vi "大富翁.vi"() -> ()   [LabVIEW 2014] (continued)
                  }
                  frame 2 {
                    n3261 = local read "玩家二財產"() -> (w2676:dbl)
                  }
                  frame 3 {
                    n3262 = local read "玩家三財產"() -> (w2677:dbl)
                  }
                  frame 4 {
                    n3263 = local read "玩家四財產"() -> (w2678:dbl)
                  }
                }
                n3264 = Equal?(x=w2622, y=w2646) -> (x = y?=w2645:bool)
                n3265 = local read "嘉義縣所有"() -> (w2623:u32)
                n3266 = local read "23旅4"() -> (w2624:bool)
                n3267 = local read "23旅3"() -> (w2625:bool)
                n3268 = local read "23旅2"() -> (w2626:bool)
                n3269 = local read "23旅1"() -> (w2627:bool)
                n3270 = local read "23房4"() -> (w2628:bool)
                n3271 = local read "23房3"() -> (w2629:bool)
                n3272 = local read "23房2"() -> (w2630:bool)
                n3273 = local read "23房1"() -> (w2631:bool)
                n3274 = call "房子數量.vi"("房子 1"=w2631, "房子 2"=w2630, "房子 3"=w2629, "房子 4"=w2628, "旅館 1"=w2627, "旅館 2"=w2626, "旅館 3"=w2625, "旅館 4"=w2624) -> ("房子數"=w2644:dbl, "旅館數"=w2643:dbl)  [unwired: 18 in]
                n3275 = call "顏色轉數字.vi"("顏色數字"=w2623) -> ("數字"=w2633:dbl)  [unwired: 2 in]
                n3276 = case shown="1, Default" w2633 {
                  tunnel: [w2651 w2652 w2653 w2654] -> w2637
                  frame 1, Default {
                    n3277 = local read "玩家一財產"() -> (w2651:dbl)
                  }
                  frame 2 {
                    n3278 = local read "玩家二財產"() -> (w2652:dbl)
                  }
                  frame 3 {
                    n3279 = local read "玩家三財產"() -> (w2653:dbl)
                  }
                  frame 4 {
                    n3280 = local read "玩家四財產"() -> (w2654:dbl)
                  }
                }
                n3281 = call "走到地.vi"("房子數量"=w2644, "自己的地?"=w2645, "旅館數量"=w2643, "編號"=w2642, "走到人財產"=w2641) -> ("走到人-?"=w2640:dbl, "蓋第幾棟"=w2638:dbl, "地主+?"=w2636:dbl, "破產?"=w2632:bool)
                n3282 = Subtract(x=w2641, y=w2640) -> (x-y=w2639:dbl)
                n3283 = Add(x=w2636, y=w2637) -> (x+y=w2634:dbl)
                n3284 = case shown="1, Default" w2633 {
                  tunnel: w2634 -> [w2647 w2648 w2649 w2650]
                  frame 1, Default {
                    n3285 = local write "玩家一財產"(w2647) -> ()
                  }
                  frame 2 {
                    n3286 = local write "玩家二財產"(w2648) -> ()
                  }
                  frame 3 {
                    n3287 = local write "玩家三財產"(w2649) -> ()
                  }
                  frame 4 {
                    n3288 = local write "玩家四財產"(w2650) -> ()
                  }
                }
                n3289 = case shown="7" w2638 {
                  frame 0, Default {
                  }
                  frame 1 {
                    n3290 = flat-sequence {
                      frame #0 {
                        n3291 = local write "23房1"(TRUE ("1房1")) -> ()
                      }
                      frame #1 {
                        n3292 = property on="23房1" class="Bool (strict)"("Visible"=TRUE) -> ()  [unwired: 2 in, 2 out]
                      }
                    }
                  }
                  frame 2 {
                    n3293 = flat-sequence {
                      frame #0 {
                        n3294 = local write "23房2"(TRUE ("1房2")) -> ()
                      }
                      frame #1 {
                        n3295 = property on="23房2" class="Bool (strict)"("Visible"=TRUE ("1房2")) -> ()  [unwired: 2 in, 2 out]
                      }
                    }
                  }
                  frame 3 {
                    n3296 = flat-sequence {
                      frame #0 {
                        n3297 = local write "23房3"(TRUE) -> ()
                      }
                      frame #1 {
                        n3298 = property on="23房3" class="Bool (strict)"("Visible"=TRUE) -> ()  [unwired: 2 in, 2 out]
                      }
                    }
                  }
                  frame 4 {
                    n3299 = flat-sequence {
                      frame #0 {
                        n3300 = local write "23房4"(TRUE) -> ()
                      }
                      frame #1 {
                        n3301 = property on="23房4" class="Bool (strict)"("Visible"=TRUE) -> ()  [unwired: 2 in, 2 out]
                      }
                    }
                  }
                  frame 5 {
                    n3302 = flat-sequence {
                      frame #0 {
                        n3303 = local write "23旅1"(TRUE) -> ()
                      }
                      frame #1 {
                        n3304 = property on="23旅1" class="Bool (strict)"("Visible"=TRUE) -> ()  [unwired: 2 in, 2 out]
                      }
                    }
                  }
                  frame 6 {
                    n3305 = flat-sequence {
                      frame #0 {
                        n3306 = local write "23旅2"(TRUE) -> ()
                      }
                      frame #1 {
                        n3307 = property on="23旅2" class="Bool (strict)"("Visible"=TRUE) -> ()  [unwired: 2 in, 2 out]
                      }
                    }
                  }
                  frame 7 {
                    n3308 = flat-sequence {
                      frame #0 {
                        n3309 = local write "23旅3"(TRUE) -> ()
                      }
                      frame #1 {
                        n3310 = property on="23旅3" class="Bool (strict)"("Visible"=TRUE) -> ()  [unwired: 2 in, 2 out]
                      }
                    }
                  }
                  frame 8 {
                    n3311 = flat-sequence {
                      frame #0 {
                        n3312 = local write "23旅4"(TRUE) -> ()
                      }
                      frame #1 {
                        n3313 = property on="23旅4" class="Bool (strict)"("Visible"=TRUE) -> ()  [unwired: 2 in, 2 out]
                      }
                    }
                  }
                }
                n3314 = case shown="1, Default" w2635 {
                  tunnel: w2639 -> [w2671 w2672 w2673 w2674]
                  frame 1, Default {
                    n3315 = local write "玩家一財產"(w2671) -> ()
                  }
                  frame 2 {
                    n3316 = local write "玩家二財產"(w2672) -> ()
                  }
                  frame 3 {
                    n3317 = local write "玩家三財產"(w2673) -> ()
                  }
                  frame 4 {
                    n3318 = local write "玩家四財產"(w2674) -> ()
                  }
                }
              }
              frame True {
                # "無主地"
                n3319 = call "購買土地.vi"() -> ("確定 2"=w2681:bool)  [unwired: 3 in]
                n3320 = case shown="True" w2681 {
                  tunnel: w2680 -> [_ w2685]
                  frame False {
                    # "不買"
                  }
                  frame True {
                    # "要買"
                    n3321 = local read "換誰?"() -> (w2686:dbl)
                    n3322 = case shown="4" w2686 {
                      tunnel: [w2713 w2714 w2715 w2716] -> w2684
                      frame 1, Default {
                        n3323 = local read "玩家一財產"() -> (w2713:dbl)
                      }
                      frame 2 {
                        n3324 = local read "玩家二財產"() -> (w2714:dbl)
                      }
                      frame 3 {
                        n3325 = local read "玩家三財產"() -> (w2715:dbl)
                      }
                      frame 4 {
                        n3326 = local read "玩家四財產"() -> (w2716:dbl)
                      }
                    }
                    n3327 = call "各種價格.vi"("Numeric"=w2685) -> ("買空地"=w2683:dbl)  [unwired: 4 in, 5 out]
                    n3328 = Greater Or Equal?(x=w2684, y=w2683) -> (x >= y?=w2682:bool)
                    n3329 = case shown="True" w2682 {
                      tunnel: w2685 -> [_ w2687]
                      frame False {
                        # "錢不夠"
                        n3330 = call "錢不夠.vi"() -> ()  [unwired: 4 in]
                      }
                      frame True {
                        # "錢夠"
                        n3331 = local read "換誰?"() -> (w2688:dbl)
                        n3332 = case shown="4" w2688 {
                          selector: w2688 -> [w2692 w2698 w2704 w2710]
                          tunnel: w2687 -> [w2691 w2697 w2703 w2709]
                          frame 1, Default {
                            # "誰買了地"
                            n3333 = call "各種價格.vi"("Numeric"=w2691) -> ("買空地"=w2690:dbl)  [unwired: 4 in, 5 out]
                            n3334 = local read "玩家一財產"() -> (w2694:dbl)
                            n3335 = Subtract(x=w2694, y=w2690) -> (x-y=w2693:dbl)
                            n3336 = local write "玩家一財產"(w2693) -> ()
                            n3337 = call "數字轉顏色.vi"("數字"=w2692) -> ("顏色數字"=w2689:dbl)  [unwired: 2 in]
                            n3338 = local write "23嘉義縣"(w2689) -> ()
                            n3339 = local write "嘉義縣所有"(w2689) -> ()
                          }
                          frame 2 {
                            # "誰買了地"
                            n3340 = call "各種價格.vi"("Numeric"=w2697) -> ("買空地"=w2696:dbl)  [unwired: 4 in, 5 out]
                            n3341 = local read "玩家二財產"() -> (w2700:dbl)
                            n3342 = Subtract(x=w2700, y=w2696) -> (x-y=w2699:dbl)
                            n3343 = local write "玩家二財產"(w2699) -> ()
                            n3344 = call "數字轉顏色.vi"("數字"=w2698) -> ("顏色數字"=w2695:dbl)  [unwired: 2 in]
                            n3345 = local write "23嘉義縣"(w2695) -> ()
                            n3346 = local write "嘉義縣所有"(w2695) -> ()
                          }
                          frame 3 {
                            # "誰買了地"
                            n3347 = local read "玩家三財產"() -> (w2705:dbl)
                            n3348 = call "各種價格.vi"("Numeric"=w2703) -> ("買空地"=w2702:dbl)  [unwired: 4 in, 5 out]
                            n3349 = Subtract(x=w2705, y=w2702) -> (x-y=w2706:dbl)
                            n3350 = call "數字轉顏色.vi"("數字"=w2704) -> ("顏色數字"=w2701:dbl)  [unwired: 2 in]
                            n3351 = local write "玩家三財產"(w2706) -> ()
                            n3352 = local write "23嘉義縣"(w2701) -> ()
                            n3353 = local write "嘉義縣所有"(w2701) -> ()
                          }
                          frame 4 {
                            # "誰買了地"
                            n3354 = call "各種價格.vi"("Numeric"=w2709) -> ("買空地"=w2708:dbl)  [unwired: 4 in, 5 out]
                            n3355 = local read "玩家四財產"() -> (w2712:dbl)
                            n3356 = Subtract(x=w2712, y=w2708) -> (x-y=w2711:dbl)
                            n3357 = local write "玩家四財產"(w2711) -> ()
                            n3358 = call "數字轉顏色.vi"("數字"=w2710) -> ("顏色數字"=w2707:dbl)  [unwired: 2 in]
                            n3359 = local write "23嘉義縣"(w2707) -> ()
                            n3360 = local write "嘉義縣所有"(w2707) -> ()
                          }
                        }
                      }
                    }
                  }
                }
              }
            }
          }
          frame 25 {
            n3361 = local read "澎湖縣所有"() -> (w2717:u32)
            n3362 = Equal?(x=w2717, y=u32 16777215) -> (x = y?=w2720:bool)
            n3363 = case shown="False" w2720 {
              tunnel: w2719 -> [w2743 w2781]
              tunnel: [w2733 FALSE] -> w2718
              frame False {
                # "有主地"
                n3364 = local read "換誰?"() -> (w2736:dbl)
                n3365 = local read "澎湖縣所有"() -> (w2724:u32)
                n3366 = call "數字轉顏色.vi"("數字"=w2736) -> ("顏色數字"=w2747:dbl)  [unwired: 2 in]
                n3367 = case shown="4" w2736 {
                  tunnel: [w2776 w2777 w2778 w2779] -> w2742
                  frame 1, Default {
                    n3368 = local read "玩家一財產"() -> (w2776:dbl)
                  }
                  frame 2 {
                    n3369 = local read "玩家二財產"() -> (w2777:dbl)
                  }
                  frame 3 {
                    n3370 = local read "玩家三財產"() -> (w2778:dbl)
                  }
                  frame 4 {
                    n3371 = local read "玩家四財產"() -> (w2779:dbl)
                  }
                }
                n3372 = Equal?(x=w2724, y=w2747) -> (x = y?=w2746:bool)
                n3373 = local read "25旅4"() -> (w2725:bool)
                n3374 = local read "25旅3"() -> (w2726:bool)
                n3375 = local read "25旅2"() -> (w2727:bool)
                n3376 = local read "25旅1"() -> (w2728:bool)
                n3377 = local read "25房4"() -> (w2729:bool)
                n3378 = local read "25房3"() -> (w2730:bool)
                n3379 = local read "25房2"() -> (w2731:bool)
                n3380 = local read "25房1"() -> (w2732:bool)
                n3381 = local read "澎湖縣所有"() -> (w2723:u32)
                n3382 = call "房子數量.vi"("房子 1"=w2732, "房子 2"=w2731, "房子 3"=w2730, "房子 4"=w2729, "旅館 1"=w2728, "旅館 2"=w2727, "旅館 3"=w2726, "旅館 4"=w2725) -> ("房子數"=w2745:dbl, "旅館數"=w2744:dbl)  [unwired: 18 in]
                n3383 = call "顏色轉數字.vi"("顏色數字"=w2723) -> ("數字"=w2734:dbl)  [unwired: 2 in]
                n3384 = case shown="1, Default" w2734 {
                  tunnel: [w2752 w2753 w2754 w2755] -> w2738
                  frame 1, Default {
                    n3385 = local read "玩家一財產"() -> (w2752:dbl)
                  }
                  frame 2 {
                    n3386 = local read "玩家二財產"() -> (w2753:dbl)
                  }
                  frame 3 {
                    n3387 = local read "玩家三財產"() -> (w2754:dbl)
                  }
                  frame 4 {
                    n3388 = local read "玩家四財產"() -> (w2755:dbl)
                  }
                }
                n3389 = call "走到地.vi"("房子數量"=w2745, "自己的地?"=w2746, "旅館數量"=w2744, "編號"=w2743, "走到人財產"=w2742) -> ("走到人-?"=w2741:dbl, "蓋第幾棟"=w2739:dbl, "地主+?"=w2737:dbl, "破產?"=w2733:bool)
                n3390 = Subtract(x=w2742, y=w2741) -> (x-y=w2740:dbl)
                n3391 = Add(x=w2737, y=w2738) -> (x+y=w2735:dbl)
                n3392 = case shown="1, Default" w2734 {
                  tunnel: w2735 -> [w2748 w2749 w2750 w2751]
                  frame 1, Default {
                    n3393 = local write "玩家一財產"(w2748) -> ()
                  }
                  frame 2 {
                    n3394 = local write "玩家二財產"(w2749) -> ()
                  }
                  frame 3 {
                    n3395 = local write "玩家三財產"(w2750) -> ()
                  }
                  frame 4 {
                    n3396 = local write "玩家四財產"(w2751) -> ()
                  }
                }
                n3397 = case shown="1" w2739 {
                  frame 0, Default {
                  }
                  frame 1 {
                    n3398 = flat-sequence {
                      frame #0 {
                        n3399 = local write "25房1"(TRUE ("1房1")) -> ()
                      }
                      frame #1 {
                        n3400 = property on="25房1" class="Bool (strict)"("Visible"=TRUE) -> ()  [unwired: 2 in, 2 out]
                      }
                    }
                  }
                  frame 2 {
                    n3401 = flat-sequence {
                      frame #0 {
                        n3402 = local write "25房2"(TRUE ("1房2")) -> ()
                      }
                      frame #1 {
                        n3403 = property on="25房2" class="Bool (strict)"("Visible"=TRUE ("1房2")) -> ()  [unwired: 2 in, 2 out]
                      }
                    }
                  }
                  frame 3 {
                    n3404 = flat-sequence {
                      frame #0 {
                        n3405 = local write "25房3"(TRUE) -> ()
                      }
                      frame #1 {
                        n3406 = property on="25房3" class="Bool (strict)"("Visible"=TRUE) -> ()  [unwired: 2 in, 2 out]
                      }
                    }
                  }
                  frame 4 {
                    n3407 = flat-sequence {
                      frame #0 {
                        n3408 = local write "25房4"(TRUE) -> ()
                      }
                      frame #1 {
                        n3409 = property on="25房4" class="Bool (strict)"("Visible"=TRUE) -> ()  [unwired: 2 in, 2 out]
                      }
                    }
                  }
                  frame 5 {
                    n3410 = flat-sequence {
                      frame #0 {
                        n3411 = local write "25旅1"(TRUE) -> ()
                      }
                      frame #1 {
                        n3412 = property on="25旅1" class="Bool (strict)"("Visible"=TRUE) -> ()  [unwired: 2 in, 2 out]
                      }
                    }
                  }
                  frame 6 {
                    n3413 = flat-sequence {
                      frame #0 {
                        n3414 = local write "25旅2"(TRUE) -> ()
                      }
                      frame #1 {
                        n3415 = property on="25旅2" class="Bool (strict)"("Visible"=TRUE) -> ()  [unwired: 2 in, 2 out]
                      }
                    }
                  }
                  frame 7 {
                    n3416 = flat-sequence {
                      frame #0 {
                        n3417 = local write "25旅3"(TRUE) -> ()
                      }
                      frame #1 {
                        n3418 = property on="25旅3" class="Bool (strict)"("Visible"=TRUE) -> ()  [unwired: 2 in, 2 out]
                      }
                    }
                  }
                  frame 8 {
                    n3419 = flat-sequence {
                      frame #0 {
                        n3420 = local write "25旅4"(TRUE) -> ()
                      }
                      frame #1 {
                        n3421 = property on="25旅4" class="Bool (strict)"("Visible"=TRUE) -> ()  [unwired: 2 in, 2 out]
                      }
                    }
                  }
                }
                n3422 = case shown="1, Default" w2736 {
                  tunnel: w2740 -> [w2772 w2773 w2774 w2775]
                  frame 1, Default {
                    n3423 = local write "玩家一財產"(w2772) -> ()
                  }
                  frame 2 {
                    n3424 = local write "玩家二財產"(w2773) -> ()
                  }
                  frame 3 {
                    n3425 = local write "玩家三財產"(w2774) -> ()
                  }
                  frame 4 {
                    n3426 = local write "玩家四財產"(w2775) -> ()
                  }
                }
              }
              frame True {
                # "無主地"
                n3427 = call "購買土地.vi"() -> ("確定 2"=w2782:bool)  [unwired: 3 in]
                n3428 = case shown="True" w2782 {
                  tunnel: w2781 -> [_ w2786]
                  frame False {
                    # "不買"
                  }
                  frame True {
                    # "要買"
                    n3429 = local read "換誰?"() -> (w2787:dbl)
                    n3430 = case shown="4" w2787 {
                      tunnel: [w2814 w2815 w2816 w2817] -> w2785
                      frame 1, Default {
                        n3431 = local read "玩家一財產"() -> (w2814:dbl)
                      }
                      frame 2 {
                        n3432 = local read "玩家二財產"() -> (w2815:dbl)
                      }
                      frame 3 {
                        n3433 = local read "玩家三財產"() -> (w2816:dbl)
                      }
                      frame 4 {
                        n3434 = local read "玩家四財產"() -> (w2817:dbl)
                      }
                    }
                    n3435 = call "各種價格.vi"("Numeric"=w2786) -> ("買空地"=w2784:dbl)  [unwired: 4 in, 5 out]
                    n3436 = Greater Or Equal?(x=w2785, y=w2784) -> (x >= y?=w2783:bool)
                    n3437 = case shown="True" w2783 {
                      tunnel: w2786 -> [_ w2788]
                      frame False {
                        # "錢不夠"
                        n3438 = call "錢不夠.vi"() -> ()  [unwired: 4 in]
                      }
                      frame True {
                        # "錢夠"
                        n3439 = local read "換誰?"() -> (w2789:dbl)
                        n3440 = case shown="2" w2789 {
                          selector: w2789 -> [w2793 w2799 w2805 w2811]
                          tunnel: w2788 -> [w2792 w2798 w2804 w2810]
                          frame 1, Default {
                            # "誰買了地"
                            n3441 = call "各種價格.vi"("Numeric"=w2792) -> ("買空地"=w2791:dbl)  [unwired: 4 in, 5 out]
                            n3442 = local read "玩家一財產"() -> (w2795:dbl)
                            n3443 = Subtract(x=w2795, y=w2791) -> (x-y=w2794:dbl)
                            n3444 = local write "玩家一財產"(w2794) -> ()
                            n3445 = call "數字轉顏色.vi"("數字"=w2793) -> ("顏色數字"=w2790:dbl)  [unwired: 2 in]
                            n3446 = local write "25澎湖縣"(w2790) -> ()
                            n3447 = local write "澎湖縣所有"(w2790) -> ()
                          }
                          frame 2 {
                            # "誰買了地"
                            n3448 = call "各種價格.vi"("Numeric"=w2798) -> ("買空地"=w2797:dbl)  [unwired: 4 in, 5 out]
                            n3449 = local read "玩家二財產"() -> (w2801:dbl)
                            n3450 = Subtract(x=w2801, y=w2797) -> (x-y=w2800:dbl)
                            n3451 = local write "玩家二財產"(w2800) -> ()
                            n3452 = call "數字轉顏色.vi"("數字"=w2799) -> ("顏色數字"=w2796:dbl)  [unwired: 2 in]
                            n3453 = local write "25澎湖縣"(w2796) -> ()
                            n3454 = local write "澎湖縣所有"(w2796) -> ()
                          }
                          frame 3 {
                            # "誰買了地"
                            n3455 = local read "玩家三財產"() -> (w2806:dbl)
                            n3456 = call "各種價格.vi"("Numeric"=w2804) -> ("買空地"=w2803:dbl)  [unwired: 4 in, 5 out]
                            n3457 = Subtract(x=w2806, y=w2803) -> (x-y=w2807:dbl)
                            n3458 = call "數字轉顏色.vi"("數字"=w2805) -> ("顏色數字"=w2802:dbl)  [unwired: 2 in]
                            n3459 = local write "玩家三財產"(w2807) -> ()
                            n3460 = local write "25澎湖縣"(w2802) -> ()
                            n3461 = local write "澎湖縣所有"(w2802) -> ()
                          }
                          frame 4 {
                            # "誰買了地"
                            n3462 = call "各種價格.vi"("Numeric"=w2810) -> ("買空地"=w2809:dbl)  [unwired: 4 in, 5 out]
                            n3463 = local read "玩家四財產"() -> (w2813:dbl)
                            n3464 = Subtract(x=w2813, y=w2809) -> (x-y=w2812:dbl)
                            n3465 = local write "玩家四財產"(w2812) -> ()
                            n3466 = call "數字轉顏色.vi"("數字"=w2811) -> ("顏色數字"=w2808:dbl)  [unwired: 2 in]
                            n3467 = local write "25澎湖縣"(w2808) -> ()
                            n3468 = local write "澎湖縣所有"(w2808) -> ()
                          }
                        }
                      }
                    }
                  }
                }
              }
            }
          }
          frame 26 {
            n3469 = local read "嘉義市所有"() -> (w2818:u32)
            n3470 = Equal?(x=w2818, y=u32 16777215) -> (x = y?=w2821:bool)
            n3471 = case shown="True" w2821 {
              tunnel: w2820 -> [w2844 w2882]
              tunnel: [w2834 FALSE] -> w2819
              frame False {
                # "有主地"
                n3472 = local read "換誰?"() -> (w2837:dbl)
                n3473 = local read "嘉義市所有"() -> (w2824:u32)
                n3474 = call "數字轉顏色.vi"("數字"=w2837) -> ("顏色數字"=w2848:dbl)  [unwired: 2 in]
                n3475 = case shown="4" w2837 {
                  tunnel: [w2877 w2878 w2879 w2880] -> w2843
                  frame 1, Default {
                    n3476 = local read "玩家一財產"() -> (w2877:dbl)
                  }
                  frame 2 {
                    n3477 = local read "玩家二財產"() -> (w2878:dbl)
                  }
                  frame 3 {
                    n3478 = local read "玩家三財產"() -> (w2879:dbl)
                  }
                  frame 4 {
                    n3479 = local read "玩家四財產"() -> (w2880:dbl)
                  }
                }
                n3480 = Equal?(x=w2824, y=w2848) -> (x = y?=w2847:bool)
                n3481 = local read "26旅4"() -> (w2826:bool)
                n3482 = local read "26旅3"() -> (w2827:bool)
                n3483 = local read "26旅2"() -> (w2828:bool)
                n3484 = local read "26旅1"() -> (w2829:bool)
                n3485 = local read "26房4"() -> (w2830:bool)
                n3486 = local read "26房3"() -> (w2831:bool)
                n3487 = local read "26房2"() -> (w2832:bool)
                n3488 = local read "26房1"() -> (w2833:bool)
                n3489 = local read "嘉義市所有"() -> (w2825:u32)
                n3490 = call "房子數量.vi"("房子 1"=w2833, "房子 2"=w2832, "房子 3"=w2831, "房子 4"=w2830, "旅館 1"=w2829, "旅館 2"=w2828, "旅館 3"=w2827, "旅館 4"=w2826) -> ("房子數"=w2846:dbl, "旅館數"=w2845:dbl)  [unwired: 18 in]
                n3491 = call "顏色轉數字.vi"("顏色數字"=w2825) -> ("數字"=w2835:dbl)  [unwired: 2 in]
                n3492 = case shown="1, Default" w2835 {
                  tunnel: [w2853 w2854 w2855 w2856] -> w2839
                  frame 1, Default {
                    n3493 = local read "玩家一財產"() -> (w2853:dbl)
                  }
                  frame 2 {
                    n3494 = local read "玩家二財產"() -> (w2854:dbl)
                  }
                  frame 3 {
                    n3495 = local read "玩家三財產"() -> (w2855:dbl)
                  }
                  frame 4 {
                    n3496 = local read "玩家四財產"() -> (w2856:dbl)
                  }
                }
                n3497 = call "走到地.vi"("房子數量"=w2846, "自己的地?"=w2847, "旅館數量"=w2845, "編號"=w2844, "走到人財產"=w2843) -> ("走到人-?"=w2842:dbl, "蓋第幾棟"=w2840:dbl, "地主+?"=w2838:dbl, "破產?"=w2834:bool)
                n3498 = Subtract(x=w2843, y=w2842) -> (x-y=w2841:dbl)
                n3499 = Add(x=w2838, y=w2839) -> (x+y=w2836:dbl)
                n3500 = case shown="1, Default" w2835 {
                  tunnel: w2836 -> [w2849 w2850 w2851 w2852]
                  frame 1, Default {
                    n3501 = local write "玩家一財產"(w2849) -> ()
                  }
                  frame 2 {
                    n3502 = local write "玩家二財產"(w2850) -> ()
                  }
                  frame 3 {
                    n3503 = local write "玩家三財產"(w2851) -> ()
                  }
                  frame 4 {
                    n3504 = local write "玩家四財產"(w2852) -> ()
                  }
                }
                n3505 = case shown="8" w2840 {
                  frame 0, Default {
                  }
                  frame 1 {
                    n3506 = flat-sequence {
                      frame #0 {
                        n3507 = local write "26房1"(TRUE ("1房1")) -> ()
                      }
                      frame #1 {
                        n3508 = property on="26房1" class="Bool (strict)"("Visible"=TRUE) -> ()  [unwired: 2 in, 2 out]
                      }
                    }
                  }
                  frame 2 {
                    n3509 = flat-sequence {
                      frame #0 {
                        n3510 = local write "26房2"(TRUE ("1房2")) -> ()
                      }
                      frame #1 {
                        n3511 = property on="26房2" class="Bool (strict)"("Visible"=TRUE ("1房2")) -> ()  [unwired: 2 in, 2 out]
                      }
                    }
                  }
                  frame 3 {
                    n3512 = flat-sequence {
                      frame #0 {
                        n3513 = local write "26房3"(TRUE) -> ()
                      }
                      frame #1 {
                        n3514 = property on="26房3" class="Bool (strict)"("Visible"=TRUE) -> ()  [unwired: 2 in, 2 out]
                      }
                    }
                  }
                  frame 4 {
                    n3515 = flat-sequence {
                      frame #0 {
                        n3516 = local write "26房4"(TRUE) -> ()
                      }
                      frame #1 {
                        n3517 = property on="26房4" class="Bool (strict)"("Visible"=TRUE) -> ()  [unwired: 2 in, 2 out]
                      }
                    }
                  }
                  frame 5 {
                    n3518 = flat-sequence {
                      frame #0 {
                        n3519 = local write "26旅1"(TRUE) -> ()
                      }
                      frame #1 {
                        n3520 = property on="26旅1" class="Bool (strict)"("Visible"=TRUE) -> ()  [unwired: 2 in, 2 out]
                      }
                    }
                  }
                  frame 6 {
                    n3521 = flat-sequence {
                      frame #0 {
                        n3522 = local write "26旅2"(TRUE) -> ()
                      }
                      frame #1 {
                        n3523 = property on="26旅2" class="Bool (strict)"("Visible"=TRUE) -> ()  [unwired: 2 in, 2 out]
                      }
                    }
                  }
                  frame 7 {
                    n3524 = flat-sequence {
                      frame #0 {
                        n3525 = local write "26旅3"(TRUE) -> ()
                      }
                      frame #1 {
                        n3526 = property on="26旅3" class="Bool (strict)"("Visible"=TRUE) -> ()  [unwired: 2 in, 2 out]
                      }
                    }
                  }
                  frame 8 {
                    n3527 = flat-sequence {
                      frame #0 {
                        n3528 = local write "26旅4"(TRUE) -> ()
                      }
                      frame #1 {
                        n3529 = property on="26旅4" class="Bool (strict)"("Visible"=TRUE) -> ()  [unwired: 2 in, 2 out]
                      }
                    }
                  }
                }
                n3530 = case shown="1, Default" w2837 {
                  tunnel: w2841 -> [w2873 w2874 w2875 w2876]
                  frame 1, Default {
                    n3531 = local write "玩家一財產"(w2873) -> ()
                  }
                  frame 2 {
                    n3532 = local write "玩家二財產"(w2874) -> ()
                  }
                  frame 3 {
                    n3533 = local write "玩家三財產"(w2875) -> ()
                  }
                  frame 4 {
                    n3534 = local write "玩家四財產"(w2876) -> ()
                  }
                }
              }
              frame True {
                # "無主地"
                n3535 = call "購買土地.vi"() -> ("確定 2"=w2883:bool)  [unwired: 3 in]
                n3536 = case shown="True" w2883 {
                  tunnel: w2882 -> [_ w2887]
                  frame False {
                    # "不買"
                  }
                  frame True {
                    # "要買"
                    n3537 = local read "換誰?"() -> (w2888:dbl)
                    n3538 = case shown="4" w2888 {
                      tunnel: [w2915 w2916 w2917 w2918] -> w2886
                      frame 1, Default {
                        n3539 = local read "玩家一財產"() -> (w2915:dbl)
                      }
                      frame 2 {
                        n3540 = local read "玩家二財產"() -> (w2916:dbl)
                      }
                      frame 3 {
                        n3541 = local read "玩家三財產"() -> (w2917:dbl)
                      }
                      frame 4 {
                        n3542 = local read "玩家四財產"() -> (w2918:dbl)
                      }
                    }
                    n3543 = call "各種價格.vi"("Numeric"=w2887) -> ("買空地"=w2885:dbl)  [unwired: 4 in, 5 out]
                    n3544 = Greater Or Equal?(x=w2886, y=w2885) -> (x >= y?=w2884:bool)
                    n3545 = case shown="True" w2884 {
                      tunnel: w2887 -> [_ w2889]
                      frame False {
                        # "錢不夠"
                        n3546 = call "錢不夠.vi"() -> ()  [unwired: 4 in]
                      }
                      frame True {
                        # "錢夠"
                        n3547 = local read "換誰?"() -> (w2890:dbl)
                        n3548 = case shown="3" w2890 {
                          selector: w2890 -> [w2894 w2900 w2906 w2912]
                          tunnel: w2889 -> [w2893 w2899 w2905 w2911]
                          frame 1, Default {
                            # "誰買了地"
                            n3549 = call "各種價格.vi"("Numeric"=w2893) -> ("買空地"=w2892:dbl)  [unwired: 4 in, 5 out]
                            n3550 = local read "玩家一財產"() -> (w2896:dbl)
                            n3551 = Subtract(x=w2896, y=w2892) -> (x-y=w2895:dbl)
                            n3552 = local write "玩家一財產"(w2895) -> ()
                            n3553 = call "數字轉顏色.vi"("數字"=w2894) -> ("顏色數字"=w2891:dbl)  [unwired: 2 in]
                            n3554 = local write "26嘉義市"(w2891) -> ()
                            n3555 = local write "嘉義市所有"(w2891) -> ()
                          }
                          frame 2 {
                            # "誰買了地"
                            n3556 = call "各種價格.vi"("Numeric"=w2899) -> ("買空地"=w2898:dbl)  [unwired: 4 in, 5 out]
                            n3557 = local read "玩家二財產"() -> (w2902:dbl)
                            n3558 = Subtract(x=w2902, y=w2898) -> (x-y=w2901:dbl)
                            n3559 = local write "玩家二財產"(w2901) -> ()
                            n3560 = call "數字轉顏色.vi"("數字"=w2900) -> ("顏色數字"=w2897:dbl)  [unwired: 2 in]
                            n3561 = local write "26嘉義市"(w2897) -> ()
                            n3562 = local write "嘉義市所有"(w2897) -> ()
                          }
                          frame 3 {
                            # "誰買了地"
                            n3563 = local read "玩家三財產"() -> (w2907:dbl)
                            n3564 = call "各種價格.vi"("Numeric"=w2905) -> ("買空地"=w2904:dbl)  [unwired: 4 in, 5 out]
                            n3565 = Subtract(x=w2907, y=w2904) -> (x-y=w2908:dbl)
                            n3566 = call "數字轉顏色.vi"("數字"=w2906) -> ("顏色數字"=w2903:dbl)  [unwired: 2 in]
                            n3567 = local write "玩家三財產"(w2908) -> ()
                            n3568 = local write "26嘉義市"(w2903) -> ()
                            n3569 = local write "嘉義市所有"(w2903) -> ()
                          }
                          frame 4 {
                            # "誰買了地"
                            n3570 = call "各種價格.vi"("Numeric"=w2911) -> ("買空地"=w2910:dbl)  [unwired: 4 in, 5 out]
                            n3571 = local read "玩家四財產"() -> (w2914:dbl)
                            n3572 = Subtract(x=w2914, y=w2910) -> (x-y=w2913:dbl)
                            n3573 = local write "玩家四財產"(w2913) -> ()
                            n3574 = call "數字轉顏色.vi"("數字"=w2912) -> ("顏色數字"=w2909:dbl)  [unwired: 2 in]
                            n3575 = local write "26嘉義市"(w2909) -> ()
                            n3576 = local write "嘉義市所有"(w2909) -> ()
                          }
                        }
                      }
                    }
                  }
                }
              }
            }
          }
          frame 27 {
            n3577 = local read "雲林縣所有"() -> (w2919:u32)
            n3578 = Equal?(x=w2919, y=u32 16777215) -> (x = y?=w2922:bool)
            n3579 = case shown="True" w2922 {
              tunnel: w2921 -> [w2945 w2983]
              tunnel: [w2935 FALSE] -> w2920
              frame False {
                # "有主地"
                n3580 = local read "換誰?"() -> (w2938:dbl)
                n3581 = local read "雲林縣所有"() -> (w2926:u32)
                n3582 = call "數字轉顏色.vi"("數字"=w2938) -> ("顏色數字"=w2949:dbl)  [unwired: 2 in]
                n3583 = case shown="4" w2938 {
                  tunnel: [w2978 w2979 w2980 w2981] -> w2944
                  frame 1, Default {
                    n3584 = local read "玩家一財產"() -> (w2978:dbl)
                  }
                  frame 2 {
                    n3585 = local read "玩家二財產"() -> (w2979:dbl)
                  }
                  frame 3 {
                    n3586 = local read "玩家三財產"() -> (w2980:dbl)
                  }
                  frame 4 {
                    n3587 = local read "玩家四財產"() -> (w2981:dbl)
                  }
                }
                n3588 = local read "雲林縣所有"() -> (w2925:u32)
                n3589 = Equal?(x=w2926, y=w2949) -> (x = y?=w2948:bool)
                n3590 = local read "27旅4"() -> (w2927:bool)
                n3591 = local read "27旅3"() -> (w2928:bool)
                n3592 = local read "27旅2"() -> (w2929:bool)
                n3593 = local read "27旅1"() -> (w2930:bool)
                n3594 = local read "27房4"() -> (w2931:bool)
                n3595 = local read "27房3"() -> (w2932:bool)
                n3596 = local read "27房2"() -> (w2933:bool)
                n3597 = local read "27房1"() -> (w2934:bool)
                n3598 = call "房子數量.vi"("房子 1"=w2934, "房子 2"=w2933, "房子 3"=w2932, "房子 4"=w2931, "旅館 1"=w2930, "旅館 2"=w2929, "旅館 3"=w2928, "旅館 4"=w2927) -> ("房子數"=w2947:dbl, "旅館數"=w2946:dbl)  [unwired: 18 in]
                n3599 = call "顏色轉數字.vi"("顏色數字"=w2925) -> ("數字"=w2936:dbl)  [unwired: 2 in]
                n3600 = case shown="1, Default" w2936 {
                  tunnel: [w2954 w2955 w2956 w2957] -> w2940
                  frame 1, Default {
                    n3601 = local read "玩家一財產"() -> (w2954:dbl)
                  }
                  frame 2 {
                    n3602 = local read "玩家二財產"() -> (w2955:dbl)
                  }
                  frame 3 {
                    n3603 = local read "玩家三財產"() -> (w2956:dbl)
                  }
                  frame 4 {
                    n3604 = local read "玩家四財產"() -> (w2957:dbl)
                  }
                }
                n3605 = call "走到地.vi"("房子數量"=w2947, "自己的地?"=w2948, "旅館數量"=w2946, "編號"=w2945, "走到人財產"=w2944) -> ("走到人-?"=w2943:dbl, "蓋第幾棟"=w2941:dbl, "地主+?"=w2939:dbl, "破產?"=w2935:bool)
                n3606 = Subtract(x=w2944, y=w2943) -> (x-y=w2942:dbl)
                n3607 = Add(x=w2939, y=w2940) -> (x+y=w2937:dbl)
                n3608 = case shown="1, Default" w2936 {
                  tunnel: w2937 -> [w2950 w2951 w2952 w2953]
                  frame 1, Default {
                    n3609 = local write "玩家一財產"(w2950) -> ()
                  }
                  frame 2 {
                    n3610 = local write "玩家二財產"(w2951) -> ()
                  }
                  frame 3 {
                    n3611 = local write "玩家三財產"(w2952) -> ()
                  }
                  frame 4 {
                    n3612 = local write "玩家四財產"(w2953) -> ()
                  }
                }
                n3613 = case shown="3" w2941 {
                  frame 0, Default {
                  }
                  frame 1 {
                    n3614 = flat-sequence {
                      frame #0 {
                        n3615 = local write "27房1"(TRUE ("1房1")) -> ()
                      }
                      frame #1 {
                        n3616 = property on="27房1" class="Bool (strict)"("Visible"=TRUE) -> ()  [unwired: 2 in, 2 out]
                      }
                    }
                  }
                  frame 2 {
                    n3617 = flat-sequence {
                      frame #0 {
                        n3618 = local write "27房2"(TRUE ("1房2")) -> ()
                      }
                      frame #1 {
                        n3619 = property on="27房2" class="Bool (strict)"("Visible"=TRUE ("1房2")) -> ()  [unwired: 2 in, 2 out]
                      }
                    }
                  }
                  frame 3 {
                    n3620 = flat-sequence {
                      frame #0 {
                        n3621 = local write "27房3"(TRUE) -> ()
                      }
                      frame #1 {
                        n3622 = property on="27房3" class="Bool (strict)"("Visible"=TRUE) -> ()  [unwired: 2 in, 2 out]
                      }
                    }
                  }
                  frame 4 {
                    n3623 = flat-sequence {
                      frame #0 {
                        n3624 = local write "27房4"(TRUE) -> ()
                      }
                      frame #1 {
                        n3625 = property on="27房4" class="Bool (strict)"("Visible"=TRUE) -> ()  [unwired: 2 in, 2 out]
                      }
                    }
                  }
                  frame 5 {
                    n3626 = flat-sequence {
                      frame #0 {
                        n3627 = local write "27旅1"(TRUE) -> ()
                      }
                      frame #1 {
                        n3628 = property on="27旅1" class="Bool (strict)"("Visible"=TRUE) -> ()  [unwired: 2 in, 2 out]
                      }
                    }
                  }
                  frame 6 {
                    n3629 = flat-sequence {
                      frame #0 {
                        n3630 = local write "27旅2"(TRUE) -> ()
                      }
                      frame #1 {
                        n3631 = property on="27旅2" class="Bool (strict)"("Visible"=TRUE) -> ()  [unwired: 2 in, 2 out]
                      }
                    }
                  }
                  frame 7 {
                    n3632 = flat-sequence {
                      frame #0 {
                        n3633 = local write "27旅3"(TRUE) -> ()
                      }
                      frame #1 {
                        n3634 = property on="27旅3" class="Bool (strict)"("Visible"=TRUE) -> ()  [unwired: 2 in, 2 out]
                      }
                    }
                  }
                  frame 8 {
                    n3635 = flat-sequence {
                      frame #0 {
                        n3636 = local write "27旅4"(TRUE) -> ()
                      }
                      frame #1 {
                        n3637 = property on="27旅4" class="Bool (strict)"("Visible"=TRUE) -> ()  [unwired: 2 in, 2 out]
                      }
                    }
                  }
                }
                n3638 = case shown="1, Default" w2938 {
                  tunnel: w2942 -> [w2974 w2975 w2976 w2977]
                  frame 1, Default {
                    n3639 = local write "玩家一財產"(w2974) -> ()
                  }
                  frame 2 {
                    n3640 = local write "玩家二財產"(w2975) -> ()
                  }
                  frame 3 {
                    n3641 = local write "玩家三財產"(w2976) -> ()
                  }
                  frame 4 {
                    n3642 = local write "玩家四財產"(w2977) -> ()
                  }
                }
              }
              frame True {
                # "無主地"
                n3643 = call "購買土地.vi"() -> ("確定 2"=w2984:bool)  [unwired: 3 in]
                n3644 = case shown="True" w2984 {
                  tunnel: w2983 -> [_ w2988]
                  frame False {
                    # "不買"
                  }
                  frame True {
                    # "要買"
                    n3645 = local read "換誰?"() -> (w2989:dbl)
                    n3646 = case shown="4" w2989 {
                      tunnel: [w3016 w3017 w3018 w3019] -> w2987
                      frame 1, Default {
                        n3647 = local read "玩家一財產"() -> (w3016:dbl)
                      }
                      frame 2 {
                        n3648 = local read "玩家二財產"() -> (w3017:dbl)
                      }
                      frame 3 {
                        n3649 = local read "玩家三財產"() -> (w3018:dbl)
                      }
                      frame 4 {
                        n3650 = local read "玩家四財產"() -> (w3019:dbl)
                      }
                    }
                    n3651 = call "各種價格.vi"("Numeric"=w2988) -> ("買空地"=w2986:dbl)  [unwired: 4 in, 5 out]
                    n3652 = Greater Or Equal?(x=w2987, y=w2986) -> (x >= y?=w2985:bool)
                    n3653 = case shown="True" w2985 {
                      tunnel: w2988 -> [_ w2990]
                      frame False {
                        # "錢不夠"
                        n3654 = call "錢不夠.vi"() -> ()  [unwired: 4 in]
                      }
                      frame True {
                        # "錢夠"
                        n3655 = local read "換誰?"() -> (w2991:dbl)
                        n3656 = case shown="1, Default" w2991 {
                          selector: w2991 -> [w2995 w3001 w3007 w3013]
                          tunnel: w2990 -> [w2994 w3000 w3006 w3012]
                          frame 1, Default {
                            # "誰買了地"
                            n3657 = call "各種價格.vi"("Numeric"=w2994) -> ("買空地"=w2993:dbl)  [unwired: 4 in, 5 out]
                            n3658 = local read "玩家一財產"() -> (w2997:dbl)
                            n3659 = Subtract(x=w2997, y=w2993) -> (x-y=w2996:dbl)
                            n3660 = local write "玩家一財產"(w2996) -> ()
                            n3661 = call "數字轉顏色.vi"("數字"=w2995) -> ("顏色數字"=w2992:dbl)  [unwired: 2 in]
                            n3662 = local write "27雲林縣"(w2992) -> ()
                            n3663 = local write "雲林縣所有"(w2992) -> ()
                          }
                          frame 2 {
                            # "誰買了地"
                            n3664 = call "各種價格.vi"("Numeric"=w3000) -> ("買空地"=w2999:dbl)  [unwired: 4 in, 5 out]
                            n3665 = local read "玩家二財產"() -> (w3003:dbl)
                            n3666 = Subtract(x=w3003, y=w2999) -> (x-y=w3002:dbl)
                            n3667 = local write "玩家二財產"(w3002) -> ()
                            n3668 = call "數字轉顏色.vi"("數字"=w3001) -> ("顏色數字"=w2998:dbl)  [unwired: 2 in]
                            n3669 = local write "27雲林縣"(w2998) -> ()
                            n3670 = local write "雲林縣所有"(w2998) -> ()
                          }
                          frame 3 {
                            # "誰買了地"
                            n3671 = local read "玩家三財產"() -> (w3008:dbl)
                            n3672 = call "各種價格.vi"("Numeric"=w3006) -> ("買空地"=w3005:dbl)  [unwired: 4 in, 5 out]
                            n3673 = Subtract(x=w3008, y=w3005) -> (x-y=w3009:dbl)
                            n3674 = call "數字轉顏色.vi"("數字"=w3007) -> ("顏色數字"=w3004:dbl)  [unwired: 2 in]
                            n3675 = local write "玩家三財產"(w3009) -> ()
                            n3676 = local write "27雲林縣"(w3004) -> ()
                            n3677 = local write "雲林縣所有"(w3004) -> ()
                          }
                          frame 4 {
                            # "誰買了地"
                            n3678 = call "各種價格.vi"("Numeric"=w3012) -> ("買空地"=w3011:dbl)  [unwired: 4 in, 5 out]
                            n3679 = local read "玩家四財產"() -> (w3015:dbl)
                            n3680 = Subtract(x=w3015, y=w3011) -> (x-y=w3014:dbl)
                            n3681 = local write "玩家四財產"(w3014) -> ()
                            n3682 = call "數字轉顏色.vi"("數字"=w3013) -> ("顏色數字"=w3010:dbl)  [unwired: 2 in]
                            n3683 = local write "27雲林縣"(w3010) -> ()
                            n3684 = local write "雲林縣所有"(w3010) -> ()
                          }
                        }
                      }
                    }
                  }
                }
              }
            }
          }
          frame 29 {
            n3685 = local read "彰化縣所有"() -> (w3020:u32)
            n3686 = Equal?(x=w3020, y=u32 16777215) -> (x = y?=w3023:bool)
            n3687 = case shown="True" w3023 {
              tunnel: w3022 -> [w3046 w3084]
              tunnel: [w3036 FALSE] -> w3021
              frame False {
                # "有主地"
                n3688 = local read "換誰?"() -> (w3039:dbl)
                n3689 = local read "彰化縣所有"() -> (w3027:u32)
                n3690 = call "數字轉顏色.vi"("數字"=w3039) -> ("顏色數字"=w3050:dbl)  [unwired: 2 in]
                n3691 = case shown="4" w3039 {
                  tunnel: [w3079 w3080 w3081 w3082] -> w3045
                  frame 1, Default {
                    n3692 = local read "玩家一財產"() -> (w3079:dbl)
                  }
                  frame 2 {
                    n3693 = local read "玩家二財產"() -> (w3080:dbl)
                  }
                  frame 3 {
                    n3694 = local read "玩家三財產"() -> (w3081:dbl)
                  }
                  frame 4 {
                    n3695 = local read "玩家四財產"() -> (w3082:dbl)
                  }
                }
                n3696 = Equal?(x=w3027, y=w3050) -> (x = y?=w3049:bool)
                n3697 = local read "彰化縣所有"() -> (w3026:u32)
                n3698 = local read "29旅4"() -> (w3028:bool)
                n3699 = local read "29旅3"() -> (w3029:bool)
                n3700 = local read "29旅2"() -> (w3030:bool)
                n3701 = local read "29旅1"() -> (w3031:bool)
                n3702 = local read "29房4"() -> (w3032:bool)
                n3703 = local read "29房3"() -> (w3033:bool)
                n3704 = local read "29房2"() -> (w3034:bool)
                n3705 = local read "29房1"() -> (w3035:bool)
                n3706 = call "房子數量.vi"("房子 1"=w3035, "房子 2"=w3034, "房子 3"=w3033, "房子 4"=w3032, "旅館 1"=w3031, "旅館 2"=w3030, "旅館 3"=w3029, "旅館 4"=w3028) -> ("房子數"=w3048:dbl, "旅館數"=w3047:dbl)  [unwired: 18 in]
                n3707 = call "顏色轉數字.vi"("顏色數字"=w3026) -> ("數字"=w3037:dbl)  [unwired: 2 in]
                n3708 = case shown="1, Default" w3037 {
                  tunnel: [w3055 w3056 w3057 w3058] -> w3041
                  frame 1, Default {
                    n3709 = local read "玩家一財產"() -> (w3055:dbl)
                  }
                  frame 2 {
                    n3710 = local read "玩家二財產"() -> (w3056:dbl)
                  }
                  frame 3 {
                    n3711 = local read "玩家三財產"() -> (w3057:dbl)
                  }
                  frame 4 {
                    n3712 = local read "玩家四財產"() -> (w3058:dbl)
                  }
                }
                n3713 = call "走到地.vi"("房子數量"=w3048, "自己的地?"=w3049, "旅館數量"=w3047, "編號"=w3046, "走到人財產"=w3045) -> ("走到人-?"=w3044:dbl, "蓋第幾棟"=w3042:dbl, "地主+?"=w3040:dbl, "破產?"=w3036:bool)
                n3714 = Subtract(x=w3045, y=w3044) -> (x-y=w3043:dbl)
                n3715 = Add(x=w3040, y=w3041) -> (x+y=w3038:dbl)
                n3716 = case shown="1, Default" w3037 {
                  tunnel: w3038 -> [w3051 w3052 w3053 w3054]
                  frame 1, Default {
                    n3717 = local write "玩家一財產"(w3051) -> ()
                  }
                  frame 2 {
                    n3718 = local write "玩家二財產"(w3052) -> ()
                  }
                  frame 3 {
                    n3719 = local write "玩家三財產"(w3053) -> ()
                  }
                  frame 4 {
                    n3720 = local write "玩家四財產"(w3054) -> ()
                  }
                }
                n3721 = case shown="0, Default" w3042 {
                  frame 0, Default {
                  }
                  frame 1 {
                    n3722 = flat-sequence {
                      frame #0 {
                        n3723 = local write "29房1"(TRUE ("1房1")) -> ()
                      }
                      frame #1 {
                        n3724 = property on="29房1" class="Bool (strict)"("Visible"=TRUE) -> ()  [unwired: 2 in, 2 out]
                      }
                    }
                  }
                  frame 2 {
                    n3725 = flat-sequence {
                      frame #0 {
                        n3726 = local write "29房2"(TRUE ("1房2")) -> ()
                      }
                      frame #1 {
                        n3727 = property on="29房2" class="Bool (strict)"("Visible"=TRUE ("1房2")) -> ()  [unwired: 2 in, 2 out]
                      }
                    }
                  }
                  frame 3 {
                    n3728 = flat-sequence {
                      frame #0 {
                        n3729 = local write "29房3"(TRUE) -> ()
                      }
                      frame #1 {
                        n3730 = property on="29房3" class="Bool (strict)"("Visible"=TRUE) -> ()  [unwired: 2 in, 2 out]
                      }
                    }
                  }
                  frame 4 {
                    n3731 = flat-sequence {
                      frame #0 {
                        n3732 = local write "29房4"(TRUE) -> ()
                      }
                      frame #1 {
                        n3733 = property on="29房4" class="Bool (strict)"("Visible"=TRUE) -> ()  [unwired: 2 in, 2 out]
                      }
                    }
                  }
                  frame 5 {
                    n3734 = flat-sequence {
                      frame #0 {
